vi "datadictionary.vi"(11 "data dictionary in":refnum<class "data bus dictionary.lvclass">) -> (2 "Value String":string, 3 "Boolean":bool)   [LabVIEW 2013, in "data bus dictionary.lvclass"]
uses:
  dictionary/data bus dictionary.lvclass
  tag/Data Type.ctl
  tag/data bus tag description.lvclass
panel:
  out "data type":T1
  out "index":i32
  in  "name":string
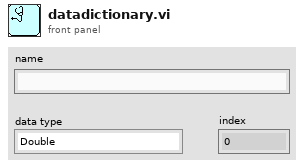
[diagram p1: front panel]
types:
  T1 = typedef "data bus tag description.lvclass/Data Type.ctl" = enum16{"Double", "I64", "Boolean", "Array of Double", "Array of I64", "Variant"}
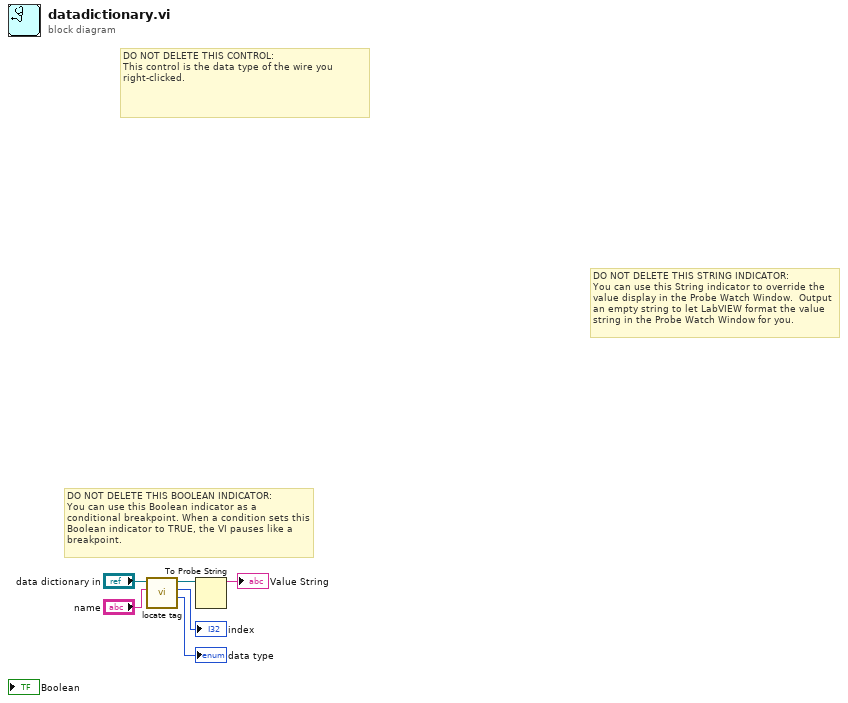
[diagram p0: block diagram]
diagram:
  # "DO NOT DELETE THIS STRING INDICATOR: \nYou can use this String indicator to override the value display in the Probe Watch Window.  Output an empty string to let LabVIEW format the value string in the Probe Watch Window for you."
  # "DO NOT DELETE THIS BOOLEAN INDICATOR: \nYou can use this Boolean indicator as a conditional breakpoint. When a condition sets this Boolean indicator to TRUE, the VI pauses like a breakpoint."
  # "DO NOT DELETE THIS CONTROL: \nThis control is the data type of the wire you right-clicked."
  n1 = call "locate tag.vi"("name"="name", "data dictionary in"="data dictionary in") -> ("data type"=→"data type":T1, "index"=→"index":i32, "data dictionary out"=w4:refnum<class "data bus dictionary.lvclass">)  [unwired: 6 in, 1 out]
  n2 = To Probe String(7:w4) -> (3:→"Value String":string)  [unwired: 2 in, 1 out]
